vi "Read Output.vi"(0 "VISA resource name":refnum<visa-resource-name>, 7 "Measurement Function (0:Voltage)":u16(ring) items=["Voltage", "Current", "Power"], 11 "error in (no error)":errorcluster) -> (4 "VISA resource name out":refnum<visa-resource-name>, 6 "Measurement":string, 15 "error out":errorcluster)   [LabVIEW 2013, in "Keithley 2200 Series.lvlib"]
doc: "Read the response from the instrument as per the selected parameter."
uses:
  Keithley 2200 Series.lvlib
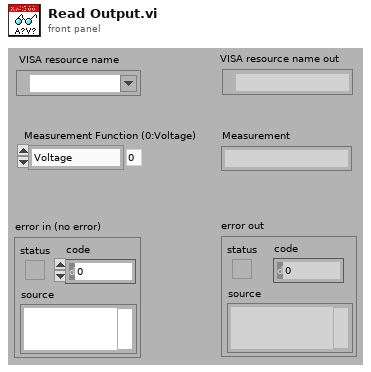
[diagram p1: front panel]
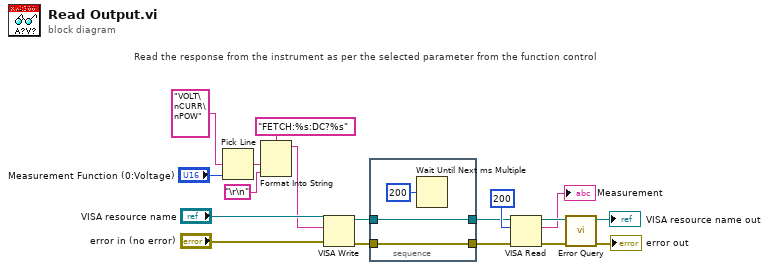
[diagram p0: block diagram]
diagram:
  # "Read the response from the instrument as per the selected parameter from the function control"
  n1 = Pick Line(multi-line string="VOLT\nCURR\nPOW" ("write buffer"), line index="Measurement Function (0:Voltage)") -> (output string=w4:string)  [unwired: 1 out]
  n2 = Format Into String(format string="FETCH:%s:DC?%s", w4, "\r\n") -> (resulting string=w1:string)  [unwired: 2 in, 1 out]
  n3 = VISA Write(VISA resource name="VISA resource name", write buffer=w1, error in (no error)="error in (no error)") -> (VISA resource name out=w11:refnum<visa-resource-name>, error out=w9:errorcluster)  [unwired: 1 out]
  n4 = stacked-sequence {
    tunnel: [w21] -> w10
    tunnel: w11 -> [w21]
    tunnel: w9 -> [w20]
    tunnel: [w20] -> w8
    frame #0 {
      n5 = Wait Until Next ms Multiple(millisecond multiple=u32 200 ("Programmable Delay in ms")) -> ()  [unwired: 1 out]
    }
  }
  n6 = VISA Read(VISA resource name=w10, byte count=u32 200, error in (no error)=w8) -> (VISA resource name out=w16:refnum<visa-resource-name>, read buffer=→"Measurement":string, error out=w15:errorcluster)  [unwired: 1 out]
  n7 = call "Error Query.vi"("error in (no error)"=w15, "VISA resource name"=w16) -> ("error out"=→"error out":errorcluster, "VISA resource name out"=→"VISA resource name out":refnum<visa-resource-name>)  [unwired: 8 out]
